vi "Entry.vi"(8 "error in (no error)":errorcluster, 11 "New State":refnum<class "Card_detection.lvclass">) -> (0 "error out":errorcluster, 3 "State out":refnum<class "Card_detection.lvclass">)   [LabVIEW 2025, in "User_Console-ATM.lvlib" / "Card_detection.lvclass"]
doc: "This is an abstract method. Override this method to define the behavior when you enter the state."
uses:
  Card_detection.lvclass
  <vilib>/ActorFramework/Actor/Actor.lvclass/Actor.ctl
  Card_detection Messages/update_card_FB Msg/update_card_FB Msg 2.lvclass/update_card_FB Msg 2.ctl
  <vilib>/ActorFramework/Message Enqueuer/Message Enqueuer.lvclass/Message Enqueuer.ctl
  <vilib>/ActorFramework/Message Enqueuer/Enqueue.vi
  Card_detection Messages/update_card_FB Msg/update_card_FB Msg 2.lvclass
  <vilib>/ActorFramework/Message Priority Queue/Priority Enqueue.vi
  User_Console_States/User_Console_States.lvclass
  Card_detection.lvclass/Card_detection.ctl
  C:/Users/halstead_rideriver/Documents/Labview_Practice/ATM_Machine_Actor Framework/ATM_ACTORFW/User_Console-ATM/User_Console_States/User_Console_States.lvclass
  C:/Program Files (x86)/National Instruments/LabVIEW 2025/vi.lib/ni/Actors/State Actor/State Actor/State Actor.lvclass
  C:/Program Files (x86)/National Instruments/LabVIEW 2025/vi.lib/ActorFramework/Actor/Actor.lvclass
  C:/Users/halstead_rideriver/Documents/Labview_Practice/ATM_Machine_Actor Framework/ATM_ACTORFW/User_Console-ATM/Card_detection/Card_detection.lvclass
  <vilib>/ActorFramework/Actor/Actor.lvclass
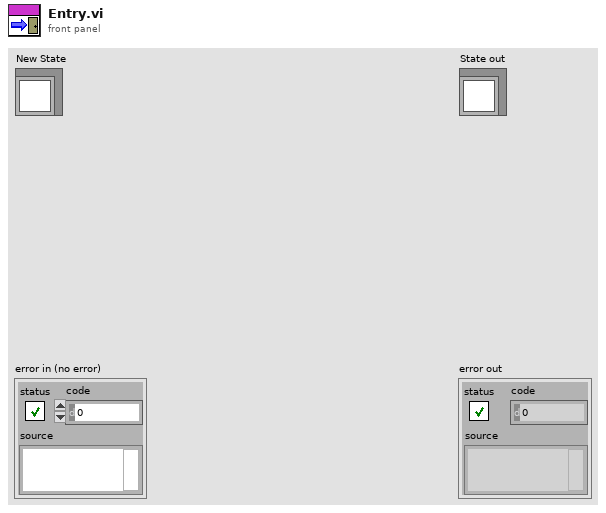
[diagram p1: front panel]
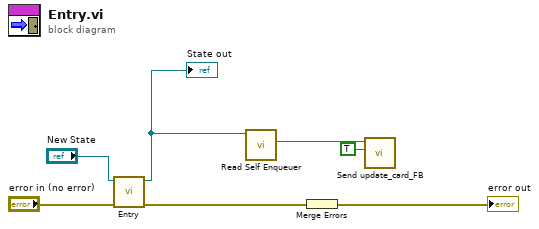
[diagram p0: block diagram]
diagram:
  n1 = call-parent "Entry.vi"("error in (no error)"="error in (no error)", "New State"="New State") -> ("error out"=w7:errorcluster, "State out"=w3:refnum<class "Card_detection.lvclass">)  [unwired: 8 in]
  "State out" <- w3
  n2 = call <vilib>:"Read Self Enqueuer.vi"("Actor"=w3) -> ("Self Enqueuer"=w2:refnum<class "Message Enqueuer.lvclass">)  [unwired: 10 in]
  n3 = Merge Errors(w7) -> (→"error out":errorcluster)
  n4 = call "Send update_card_FB.vi"("Card"=TRUE, "Message Enqueuer"=w2) -> ()  [unwired: 8 in, 2 out]
